vi "reshapeArray_FGV.vi"(6 "single image size":i32, 7 "command":T1=enum."read", 8 "error in (no error)":errorcluster, 9 "reshapedArray CamX":dbl[](array[numeric]), 10 "index":i32, 11 "emptyImageArray":dbl[](array[numeric])) -> (0 "error in (no error) 2":errorcluster, 3 "ImageArray":dbl[](array[numeric]))   [LabVIEW 2011]
uses:
  reshapeArrayCommand_TypDEf.ctl
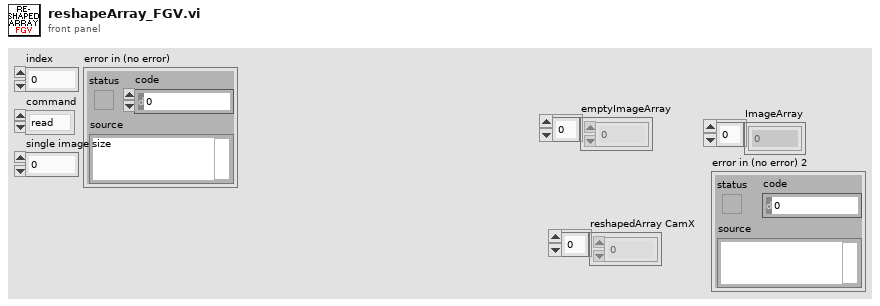
[diagram p1: front panel]
types:
  T1 = typedef "reshapeArrayCommand_TypDEf.ctl" = enum16{"init array", "addImage", "read", "init resolution"}
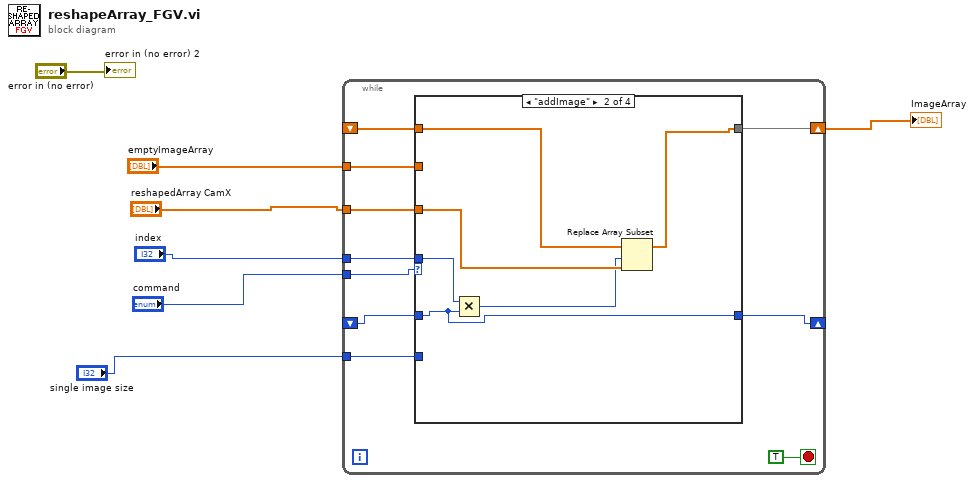
[diagram p0: block diagram]
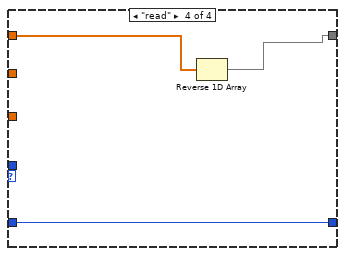
[diagram p4: hidden frame]
diagram:
  n1 = while {
    tunnel: "command" -> [w17]
    tunnel: "emptyImageArray" -> [w16]
    shift-right: [w15] -> w3
    shift-left: _ -> [w14]
    tunnel: "reshapedArray CamX" -> [w12]
    tunnel: "index" -> [w13]
    tunnel: "single image size" -> [w11]
    shift-right: [w9] -> _
    shift-left: _ -> [w8]
    stop <- TRUE stop-if-true
    n2 = case shown="\"addImage\"" w17 {
      tunnel: w16 -> [w19 _ _ _]
      tunnel: [w19 w21 w27 w29] -> w15
      tunnel: w14 -> [_ w25 w27 w30]
      tunnel: w13 -> [_ w23 _ _]
      tunnel: w12 -> [_ w24 _ _]
      tunnel: w11 -> [_ _ w26 _]
      tunnel: [w18 w20 w26 w28] -> w9
      tunnel: w8 -> [w18 w20 _ w28]
      frame "init array", Default {
      }
      frame "addImage" {
        n3 = Multiply(x=w23, y=w20) -> (x*y=w22:i32)
        n4 = Replace Array Subset(array=w25, new element=w24, index=w22) -> (w21:dbl[])
      }
      frame "init resolution" {
      }
      frame "read" {
        n5 = Reverse 1D Array(array=w30) -> (reversed array=w29:dbl[])
      }
    }
  }
  "ImageArray" <- w3
  "error in (no error) 2" <- "error in (no error)"
